vi "Log Debug Event.vi"(8 "error in (no error)":errorcluster, 10 "Debug Data.lvclass":refnum<class "Debug Data.lvclass">, 11 "Debugger in":refnum<class "Debugger.lvclass">) -> (0 "error out":errorcluster, 3 "Debugger out":refnum<class "Debugger.lvclass">)   [LabVIEW 2020, in "Debugger.lvclass"]
uses:
  Debugger.lvclass
  Debug Data/Debug Data.lvclass
  Debugger.lvclass/Debugger.ctl
  Debug Log/Debug Log.lvclass
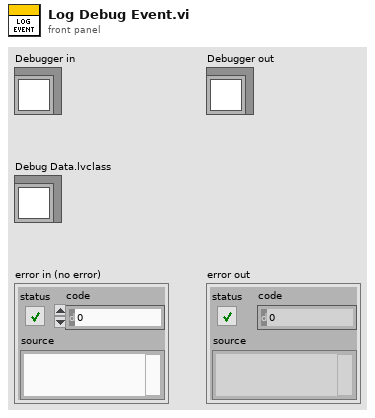
[diagram p1: front panel]
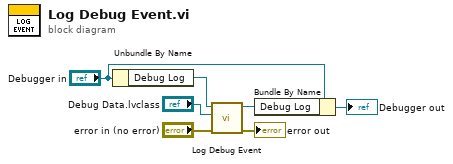
[diagram p0: block diagram]
diagram:
  n1 = Unbundle By Name("Debugger in") -> ("Debug Log"=w5:refnum<class "Debug Log.lvclass">)
  n2 = call "Log Debug Event.vi"("error in (no error)"="error in (no error)", "Debug Data.lvclass"="Debug Data.lvclass", "Debugger in"=w5) -> ("error out"=→"error out":errorcluster, "Debugger out"=w4:refnum<class "Debug Log.lvclass">)  [unwired: 7 in]
  n3 = Bundle By Name(cluster="Debugger in", "Debug Log"=w4) -> (→"Debugger out":refnum<class "Debugger.lvclass">)
